vi "measVoltGlobVarsWrite.vi"(0 "measVoltPulseLength(25ns)":i32, 2 "measVoltTimeout(10ns)":i32 caption="measVoltTimeout(25ns)", 4 "timedOutWhileHandshake":bool, 5 "measVoltState":T1, 10 "writeOnlyMeasVoltState":bool) -> ()   [LabVIEW 2014]
uses:
  Controls/measVoltState.ctl
  <vilib>/rvi/Emulation/niFpgaSctlEmulationGetInTimedLoop.vi
  measVoltGlobVars.vi
  <vilib>/rvi/Emulation/niFpgaProcessEmulError.vi
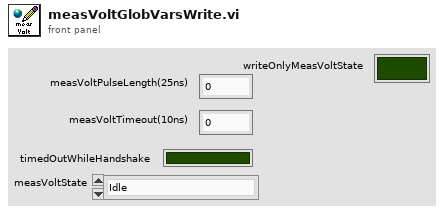
[diagram p1: front panel]
types:
  T1 = typedef "measVoltState.ctl" = enum16{"Idle", "sendMeasRequest", "waitUntilDone", "done"}
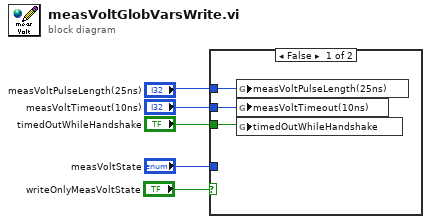
[diagram p0: block diagram]
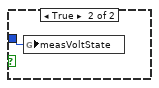
[diagram p2: hidden frame]
diagram:
  n1 = case shown="False" "writeOnlyMeasVoltState" {
    tunnel: "measVoltState" -> [_ w9]
    tunnel: "timedOutWhileHandshake" -> [w8 _]
    tunnel: "measVoltTimeout(10ns)" -> [w7 _]
    tunnel: "measVoltPulseLength(25ns)" -> [w6 _]
    frame False {
      n2 = global write "measVoltGlobVars.vi" "measVoltPulseLength(25ns)"(w6) -> ()
      n3 = global write "measVoltGlobVars.vi" "measVoltTimeout(10ns)"(w7) -> ()
      n4 = global write "measVoltGlobVars.vi" "timedOutWhileHandshake"(w8) -> ()
    }
    frame True {
      n5 = global write "measVoltGlobVars.vi" "measVoltState"(w9) -> ()
    }
  }
